vi "Write Setpoints.vi"(10 "Setpoints":T1[](array[typedef]), 11 "Temperature Control in":refnum<class "Temperature Control.lvclass">) -> (3 "Temperature Control out":refnum<class "Temperature Control.lvclass">)   [LabVIEW 2020, in "Temperature Control.lvclass"]
uses:
  Temperature Control.lvclass
  Controls/Set point.ctl
  Temperature Control.lvclass/Temperature Control.ctl
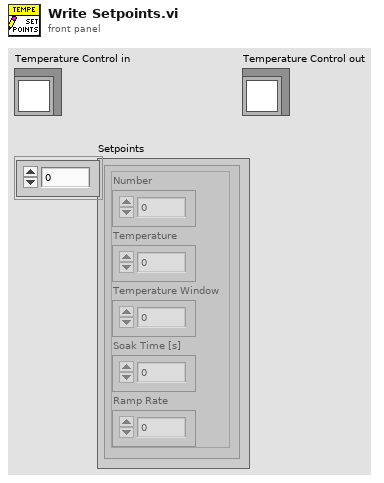
[diagram p1: front panel]
types:
  T1 = typedef "Temperature Control.lvclass/Set point.ctl" = cluster{"Number":u32, "Temperature":dbl, "Temperature Window":dbl, "Soak Time [s]":u32, "Ramp Rate":dbl}
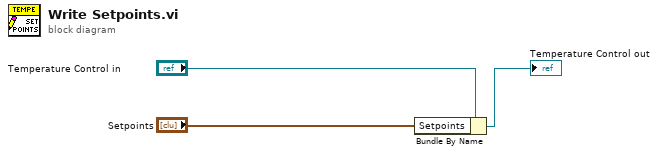
[diagram p0: block diagram]
diagram:
  n1 = Bundle By Name(cluster="Temperature Control in", "Setpoints"="Setpoints") -> (→"Temperature Control out":refnum<class "Temperature Control.lvclass">)
